vi "Write FunctionSetHandlerLevel.vi"(8 "error in (no error)":errorcluster, 10 "FunctionSetHandlerLevel":string, 11 "Handler in":refnum<class "Handler.lvclass">) -> (0 "error out":errorcluster, 3 "Handler out":refnum<class "Handler.lvclass">)   [LabVIEW 2022 SP3, in "Logger.lvlib" / "Handler.lvclass"]
uses:
  Handler.lvclass
  Handler.lvclass/Handler.ctl
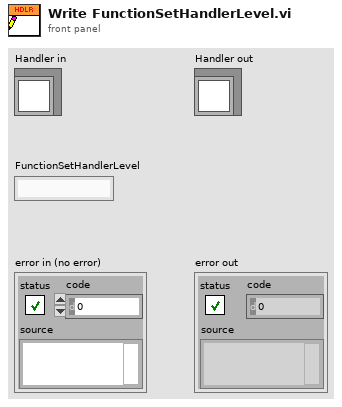
[diagram p1: front panel]
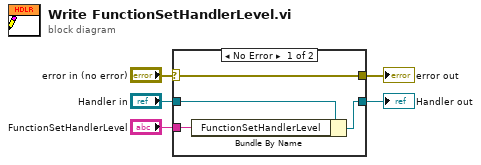
[diagram p0: block diagram]
diagram:
  n1 = case shown="No Error" "error in (no error)" {
    selector: "error in (no error)" -> [w9 w10]
    tunnel: [w9 w10] -> w4
    tunnel: [w7 w11] -> w2
    tunnel: "Handler in" -> [w8 w11]
    tunnel: "FunctionSetHandlerLevel" -> [w6 _]
    frame No Error {
      n2 = Bundle By Name(cluster=w8, "FunctionSetHandlerLevel"=w6) -> (w7:refnum<class "Handler.lvclass">)
    }
    frame Error {
    }
  }
  "error out" <- w4
  "Handler out" <- w2
